vi "Create Logger.vi"(7 "framework options":T1, 8 "error in (no error)":errorcluster, 10 "log file directory":path, 11 "Framework in":refnum<class "Framework.lvclass">) -> (0 "error out":errorcluster, 1 "Logging Interface":refnum<class "Logging Interface.lvclass">, 2 "Logging Thread":refnum<class "Logging Thread.lvclass">, 3 "Framework out":refnum<class "Framework.lvclass">)   [LabVIEW 2017, in "DSF Core.lvlib" / "Framework.lvclass"]
uses:
  Framework.lvclass
  Thread/Logging/Logging Thread.lvclass
  Framework Options.ctl
  Typedefs/DSF FIFO Options.ctl
  Thread/DSF Thread Options.ctl
  Typedefs/DSF Plugin Options.ctl
  Typedefs/DSF Performance Options.ctl
  Interface/Logging/Logging Interface.lvclass
  Thread/Thread Settings.ctl
  Framework.lvclass/Framework.ctl
  Thread/Thread.lvclass
  DSF Core.lvlib
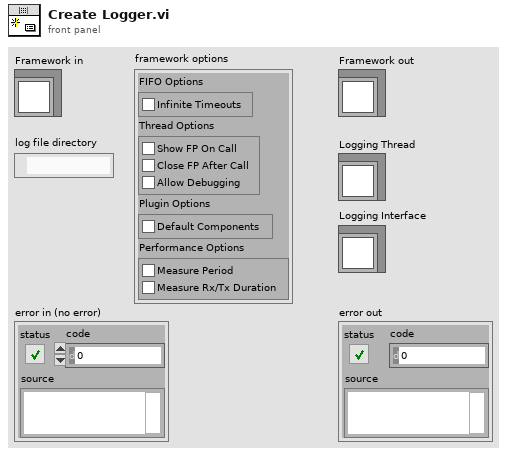
[diagram p1: front panel]
types:
  T1 = typedef "DSF Core.lvlib/Framework.lvclass/Framework Options.ctl" = cluster{"FIFO Options":T2, "Thread Options":T3, "Plugin Options":T4, "Performance Options":T5}
  T2 = typedef "DSF Core.lvlib/DSF FIFO Options.ctl" = cluster{"Infinite Timeouts":bool}
  T3 = typedef "DSF Core.lvlib/DSF Thread Options.ctl" = cluster{"Show FP On Call":bool, "Close FP After Call":bool, "Allow Debugging":bool}
  T4 = typedef "DSF Core.lvlib/DSF Plugin Options.ctl" = cluster{"Default Components":bool}
  T5 = typedef "DSF Core.lvlib/DSF Performance Options.ctl" = cluster{"Measure Period":bool, "Measure Rx/Tx Duration":bool}
  T6 = typedef "DSF Core.lvlib/Thread.lvclass/Thread Settings.ctl" = cluster{"Priority":u16, "Processor":i32, "ID":i32}
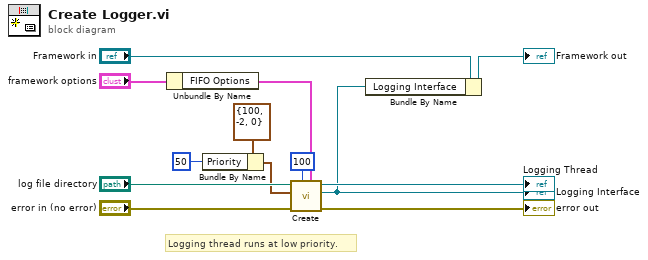
[diagram p0: block diagram]
diagram:
  # "Logging thread runs at low priority."
  n1 = Unbundle By Name("framework options") -> ("FIFO Options"=w5:T2)
  n2 = Bundle By Name(cluster=T6 {"Priority"=100, "Processor"=-2, "ID"=0} ("Thread Parameters"), "Priority"=u16 50 ("priority (100)")) -> (w1:T6)
  n3 = call "Create.vi"("FIFO Options"=w5, "fifo depths (100)"=u32 100 ("fifo depths"), "error in (no error)"="error in (no error)", "thread settings"=w1, "log file directory"="log file directory") -> ("error out"=→"error out":errorcluster, "Logging Interface"=w3:refnum<class "Logging Interface.lvclass">, "Logging Thread out"=→"Logging Thread":refnum<class "Logging Thread.lvclass">)  [unwired: 4 in]
  "Logging Interface" <- w3
  n4 = Bundle By Name(cluster="Framework in", "Logging Interface"=w3) -> (→"Framework out":refnum<class "Framework.lvclass">)
